vi "Read Last Controlword.vi"(8 "error in (no error)":errorcluster, 11 "Motor Base in":refnum<class "Motor Base.lvclass">) -> (0 "error out":errorcluster, 2 "Controlword":string(combo), 3 "Motor Base out":refnum<class "Motor Base.lvclass">)   [LabVIEW 2016, in "Motor Base.lvlib" / "Motor Base.lvclass"]
uses:
  Motor Base.lvclass
  Motor Base.lvclass/Motor Base.ctl
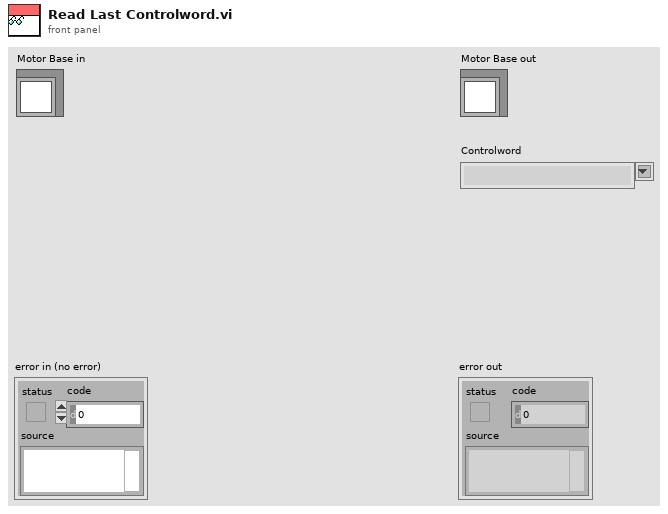
[diagram p1: front panel]
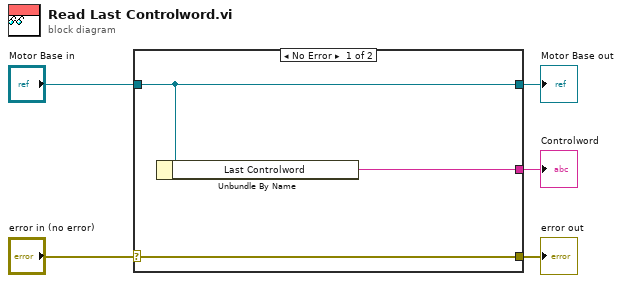
[diagram p0: block diagram]
diagram:
  n1 = case shown="No Error" "error in (no error)" {
    selector: "error in (no error)" -> [w8 w9]
    tunnel: [w8 w9] -> w4
    tunnel: [w7 w10] -> w2
    tunnel: "Motor Base in" -> [w7 w10]
    tunnel: [w6 _] -> w1
    frame No Error {
      n2 = Unbundle By Name(w7) -> ("Last Controlword"=w6:string)
    }
    frame Error {
    }
  }
  "error out" <- w4
  "Motor Base out" <- w2
  "Controlword" <- w1
